vi "Process.vi"(11 "AI Manager in":refnum<class "AI Manager.lvclass">) -> (1 "Velocity out":dbl, 2 "Direction out":cluster{dbl, dbl}, 4 "Self Index out":i32, 5 "Boost ?":bool)   [LabVIEW 2021, in "AI Manager.lvclass"]
doc: "MIT Licence\nCopyright (c) 2024 David Grollier"
uses:
  AI Manager.lvclass
  AI Manager.lvclass/AI Manager.ctl
  Game Componants/Game Componants.lvclass/Game Componants.ctl
  Game Componants/Game Board Component/Movable/Movable.lvclass
  C:/Users/David/Documents/GameSoccerSpace/Source/Game Componants/Game Componants.lvclass
  Game Componants/Game Board Component/Movable/Flying Saucer/Flying Saucer.lvclass
  Game Componants/Game Componants.lvclass
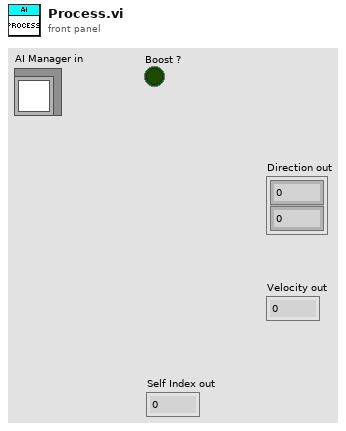
[diagram p1: front panel]
types:
  T1 = typedef "Coordinates.ctl" = cluster{"x":dbl, "y":dbl}
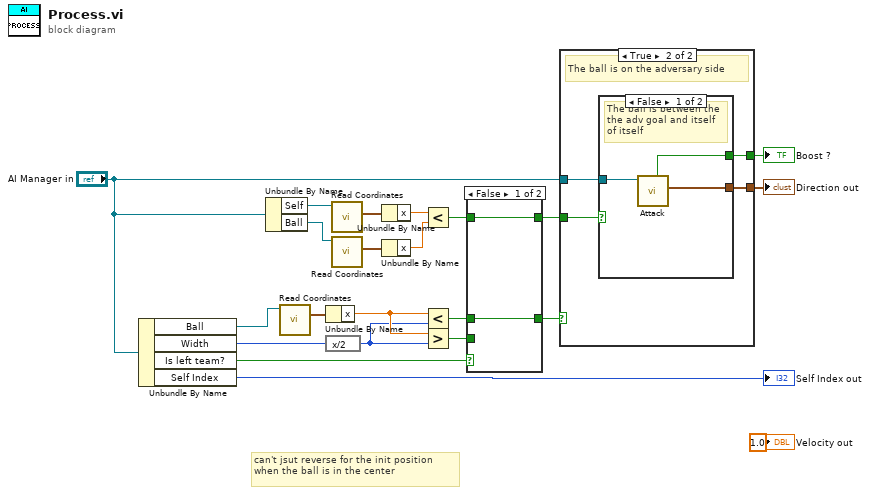
[diagram p0: block diagram]
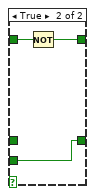
[diagram p2: hidden frame]
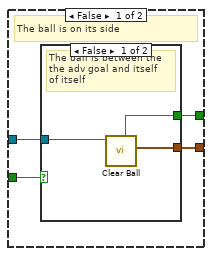
[diagram p3: hidden frame]
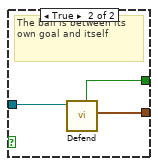
[diagram p4: hidden frame]
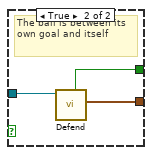
[diagram p5: hidden frame]
diagram:
  # "can't jsut reverse for the init position when the ball is in the center"
  n1 = Unbundle By Name("AI Manager in") -> ("Ball"=w20:refnum<class "Movable.lvclass">, "Width"=w21:u32, "Is left team?"=w12:bool, "Self Index"=→"Self Index out":i32)
  n2 = Unbundle By Name("AI Manager in") -> ("Self"=w13:refnum<class "Flying Saucer.lvclass">, "Ball"=w18:refnum<class "Movable.lvclass">)
  n3 = call "Read Coordinates.vi"("Game Componants in"=w20) -> ("Coordinates"=w19:T1)  [unwired: 10 in]
  n4 = Unbundle By Name(w19) -> ("x"=w7:dbl)
  n5 = expression code="x/2"(w21) -> (w6:u32)
  n6 = call "Read Coordinates.vi"("Game Componants in"=w13) -> ("Coordinates"=w17:T1)  [unwired: 10 in]
  n7 = call "Read Coordinates.vi"("Game Componants in"=w18) -> ("Coordinates"=w16:T1)  [unwired: 10 in]
  n8 = Unbundle By Name(w17) -> ("x"=w14:dbl)
  n9 = Unbundle By Name(w16) -> ("x"=w15:dbl)
  n10 = Less?(x=w14, y=w15) -> (x < y?=w10:bool)
  n11 = Less?(x=w7, y=w6) -> (x < y?=w8:bool)
  n12 = Greater?(x=w7, y=w6) -> (0:w5:bool)
  n13 = case shown="False" w12 {
    tunnel: [w24 w26] -> w11
    tunnel: w10 -> [w24 w27]
    tunnel: [w23 w25] -> w9
    tunnel: w8 -> [w23 _]
    tunnel: w5 -> [_ w25]
    frame False {
    }
    frame True {
      n14 = Not(x=w27) -> (.not. x?=w26:bool)
    }
  }
  n15 = case shown="True" w9 {
    tunnel: "AI Manager in" -> [w31 w41]
    tunnel: [w30 w40] -> w2
    tunnel: [w29 w39] -> w3
    tunnel: w11 -> [w28 w38]
    frame False {
      # "The ball is on its side"
      n16 = case shown="False" w28 {
        tunnel: w31 -> [w34 w37]
        tunnel: [w33 w36] -> w30
        tunnel: [w32 w35] -> w29
        frame False {
          # "The ball is between the the adv goal and itself\nof itself"
          n17 = call "Clear Ball.vi"("AI Manager in"=w34) -> ("Direction out"=w32:cluster{dbl, dbl}, "Boost?"=w33:bool)  [unwired: 9 in]
        }
        frame True {
          # "The ball is between its own goal and itself"
          n18 = call "Defend.vi"("AI Manager in"=w37) -> ("Direction out"=w35:cluster{dbl, dbl}, "Boost ?"=w36:bool)  [unwired: 9 in]
        }
      }
    }
    frame True {
      # "The ball is on the adversary side"
      n19 = case shown="False" w38 {
        tunnel: w41 -> [w44 w47]
        tunnel: [w43 w46] -> w40
        tunnel: [w42 w45] -> w39
        frame False {
          # "The ball is between the the adv goal and itself\nof itself"
          n20 = call "Attack.vi"("AI Manager in"=w44) -> ("Direction out"=w42:cluster{dbl, dbl}, "Boost ?"=w43:bool)  [unwired: 9 in]
        }
        frame True {
          # "The ball is between its own goal and itself"
          n21 = call "Defend.vi"("AI Manager in"=w47) -> ("Direction out"=w45:cluster{dbl, dbl}, "Boost ?"=w46:bool)  [unwired: 9 in]
        }
      }
    }
  }
  "Direction out" <- w3
  "Boost ?" <- w2
  "Velocity out" <- 1.0 ("Velocity out")
